vi "Continuous_Measurement_v3.vi"() -> ()   [LabVIEW 2014]
uses:
  <vilib>/Analysis/NI_AALBase.lvlib
panel:
  out "Start Timer":u32
  out "I":dbl[](array[numeric])
  out "V":dbl[](array[numeric])
  out "T":dbl[](array[numeric])
  out "File Startname":string
  in  "stop":bool
  out "I-t Graph":cluster{u32[], "I":dbl[]}(graph)
  out "V-t Graph":cluster{u32[], "V":dbl[]}(graph)
  out "V-I Graph":cluster{dbl[], dbl[]}(graph)
  in  "Meas. wait time (ms)":i32
  in  "Meas. to Avg":i32
  out "Voltage (V)":string
  in  "Current (uA)":dbl
  in  "Collect":bool
  in  "Outp. wait time (ms)":i32
  in  "2182A VISA":refnum<visa-resource-name>
  in  "Output Response":bool
  in  "Compliance (V)":dbl
  out "File Counter":i32
  out "Data Counter":i32
  in  "6221 VISA":refnum<visa-resource-name>
  in  "First Path":path
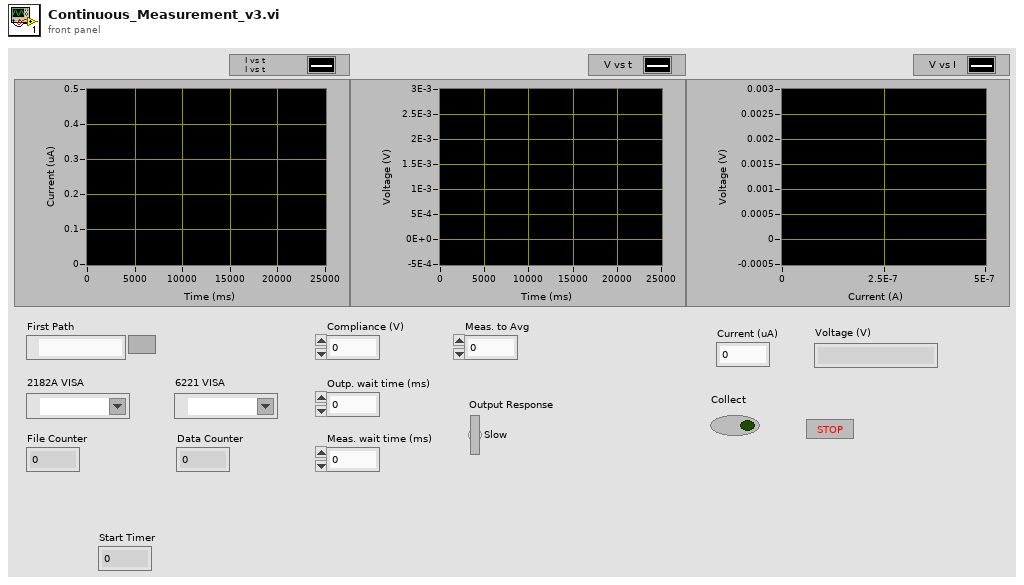
[diagram p1: front panel]
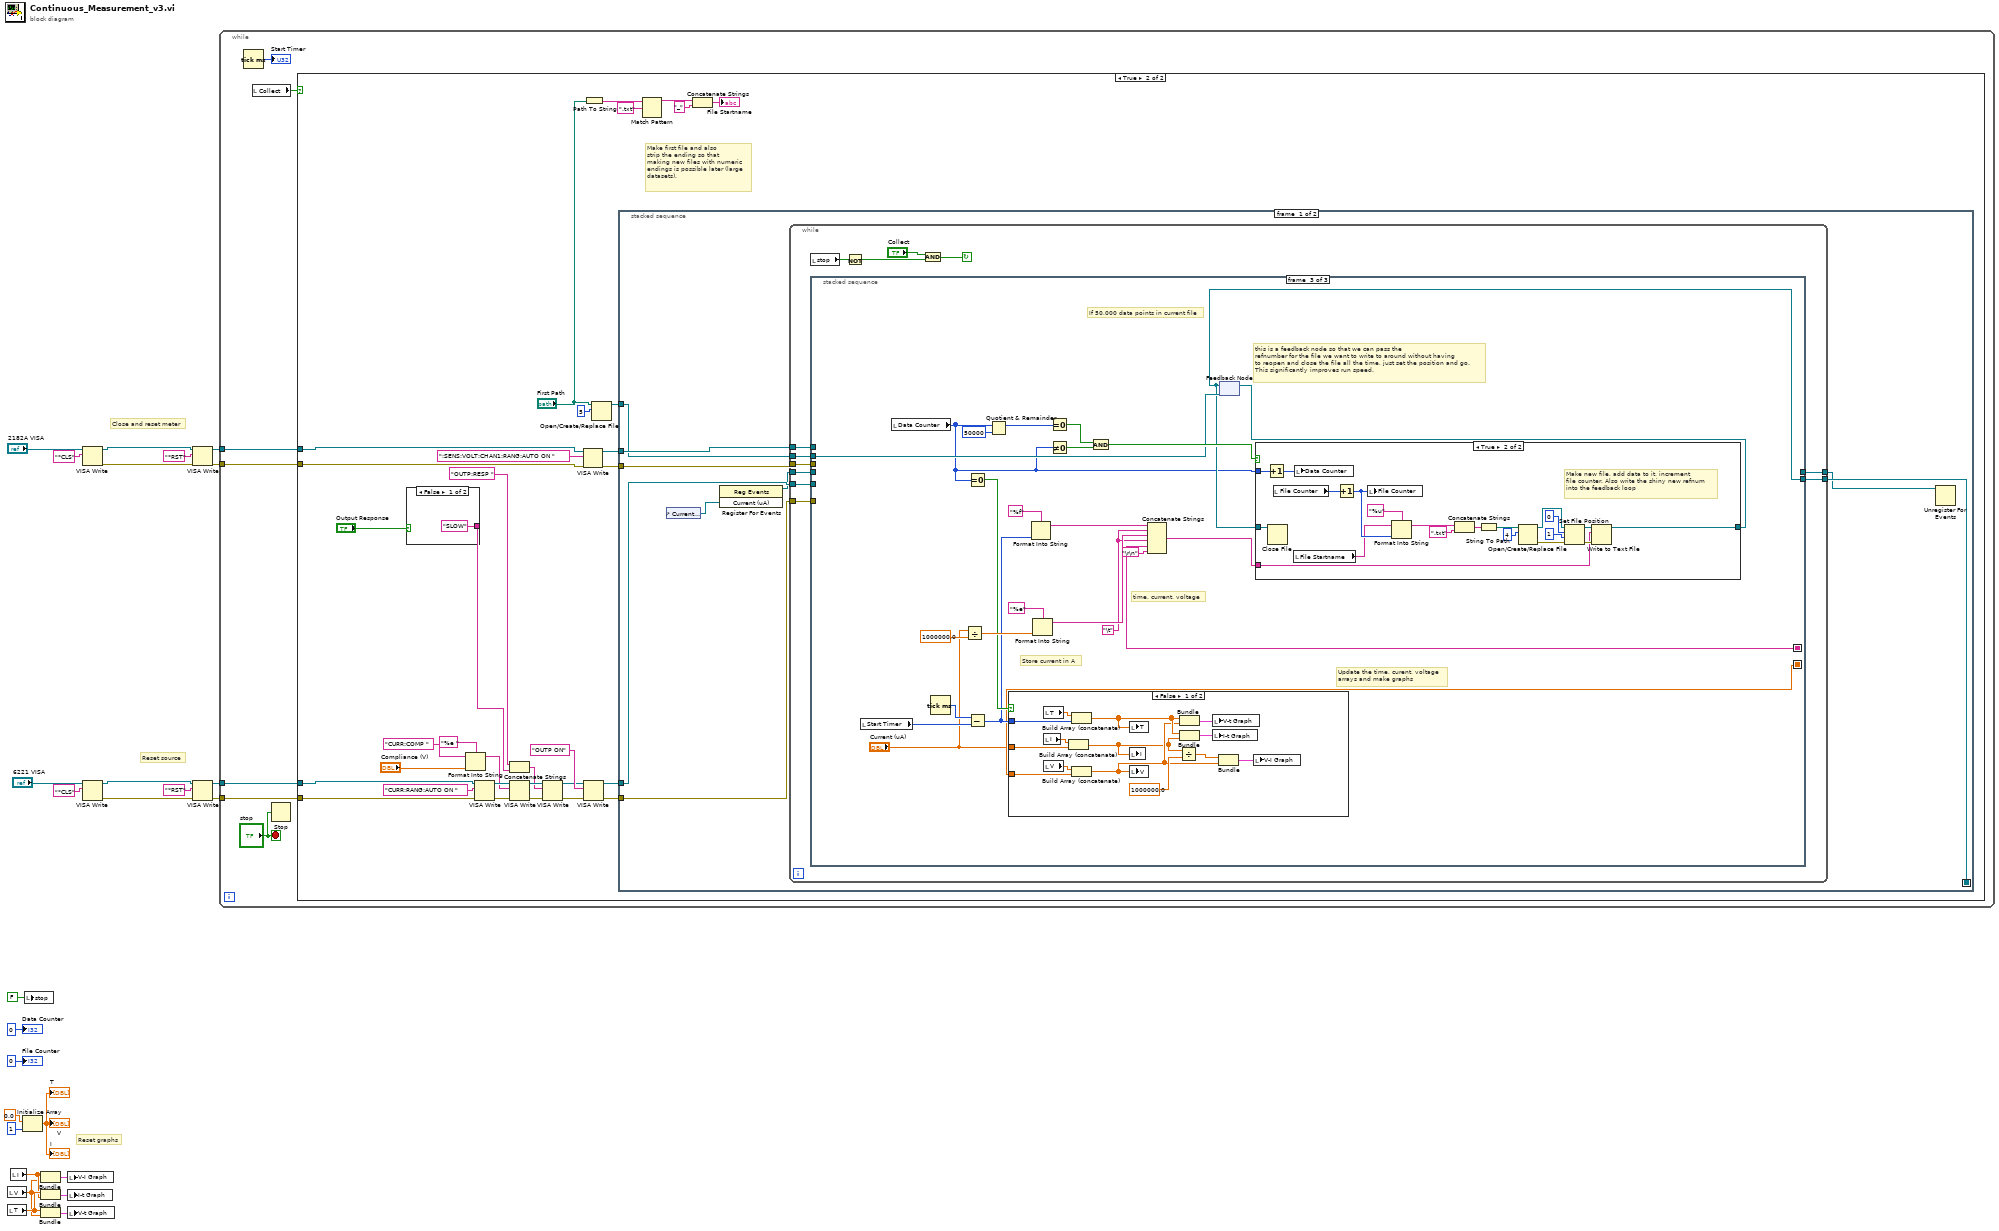
[diagram p0: block diagram]
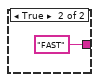
[diagram p3: hidden frame]
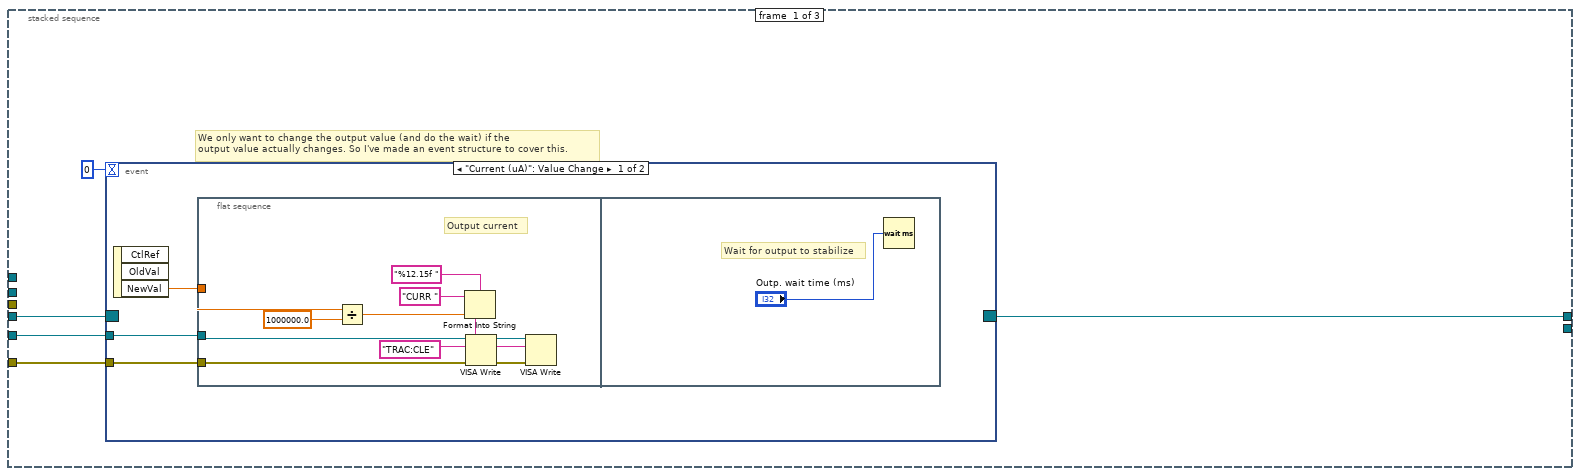
[diagram p4: hidden frame]
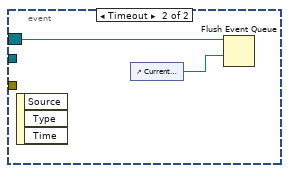
[diagram p5: hidden frame]
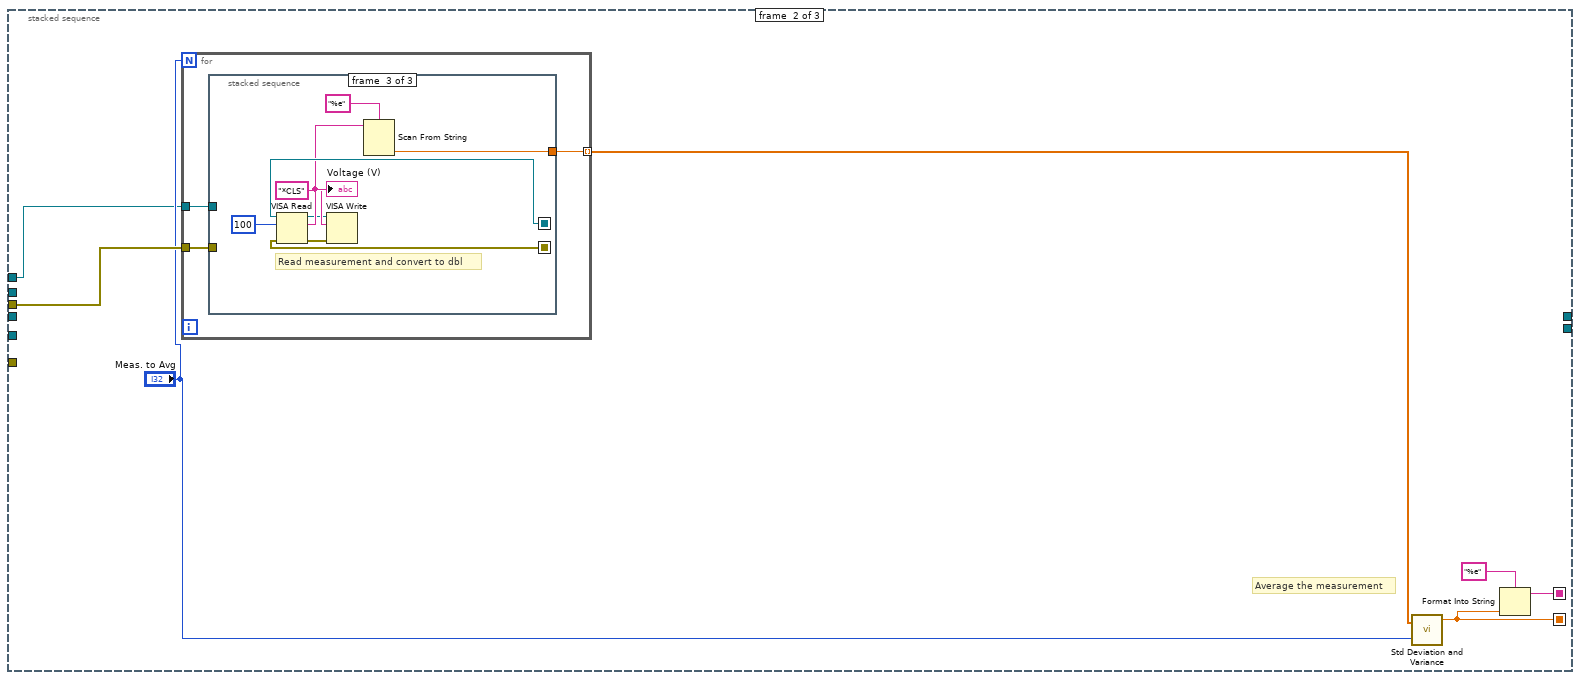
[diagram p6: hidden frame]
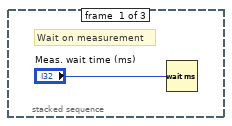
[diagram p7: hidden frame]
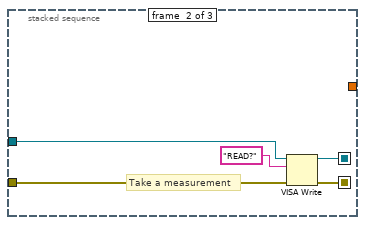
[diagram p8: hidden frame]
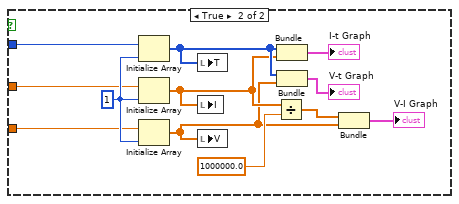
[diagram p9: hidden frame]
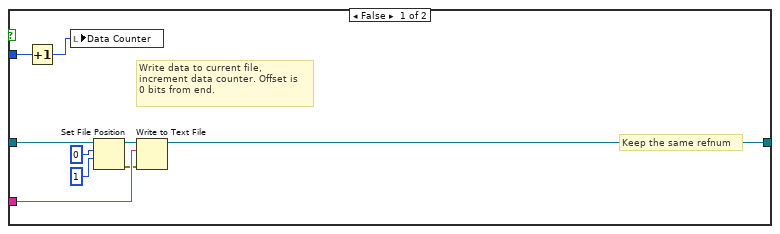
[diagram p10: hidden frame]
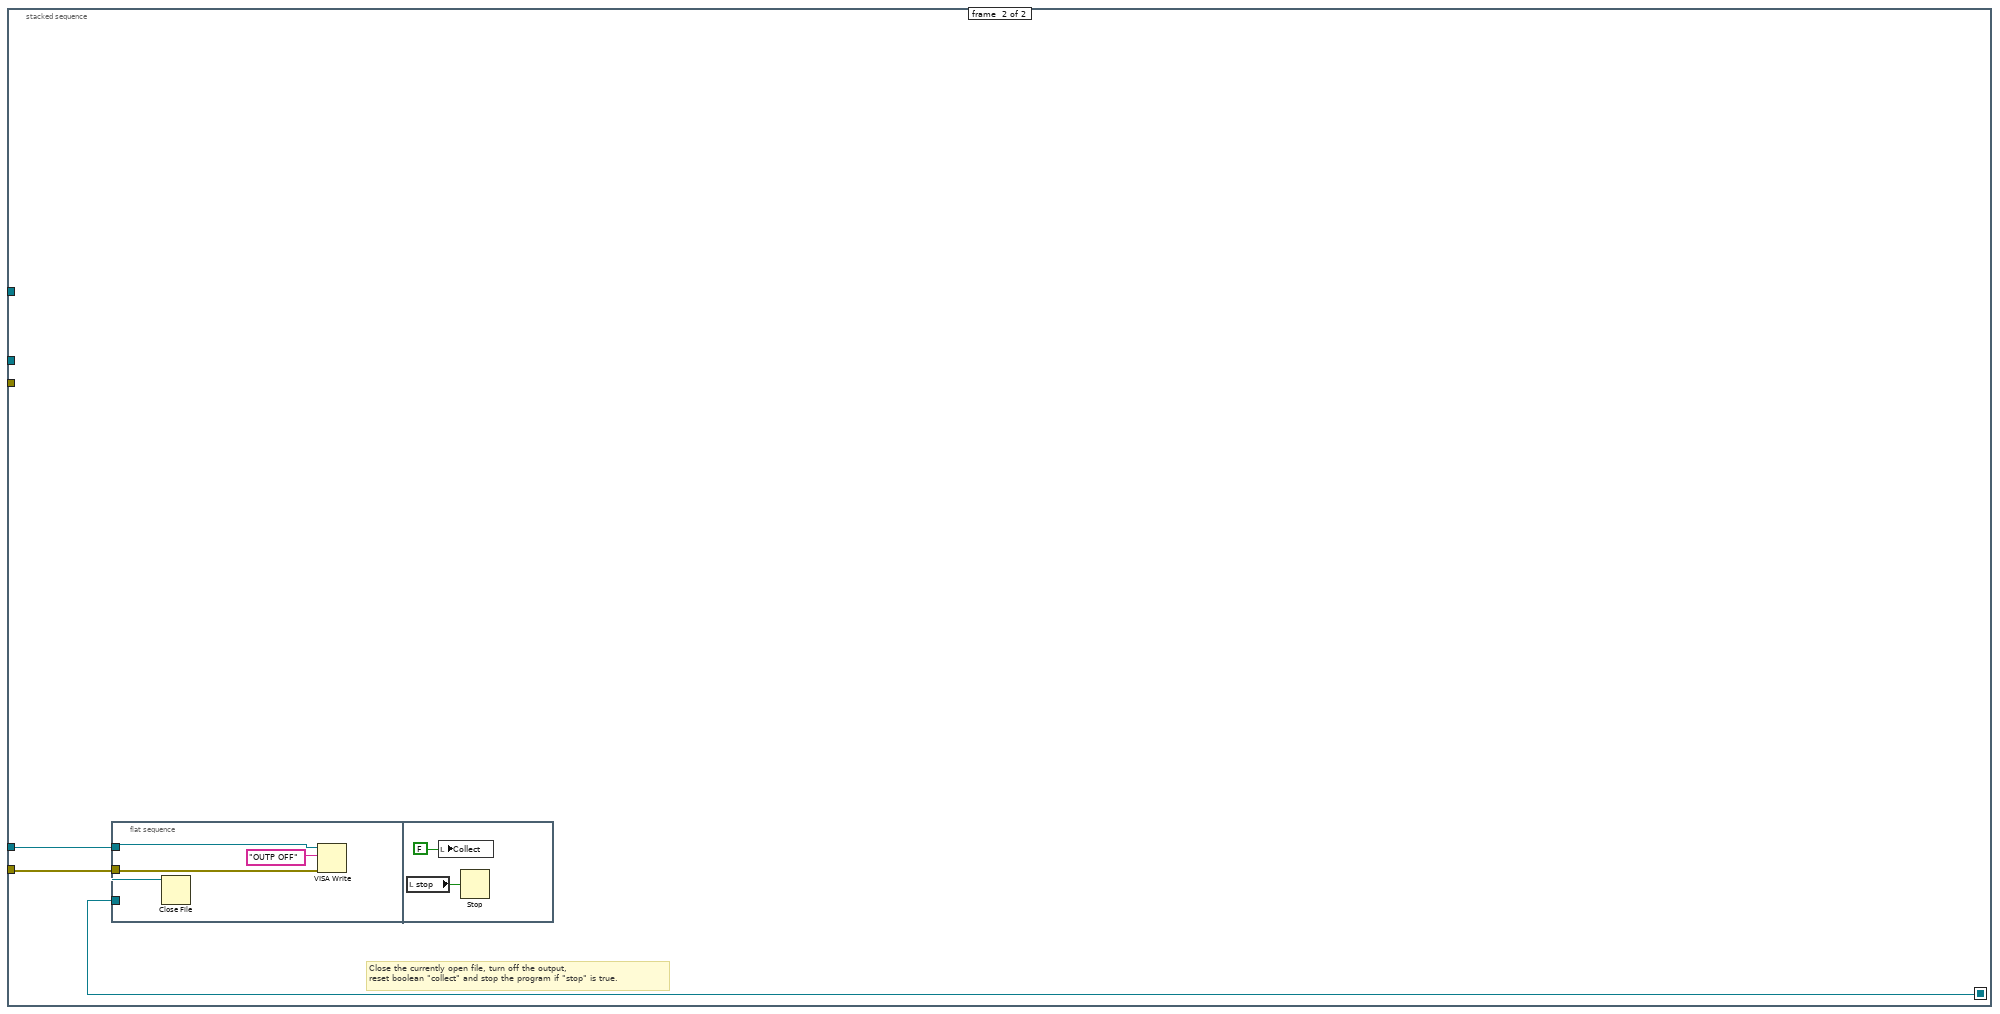
[diagram p11: hidden frame]
diagram:
  # "Reset graphs"
  # "Reset source"
  # "Close and reset meter"
  n1 = local read "V"() -> (w4:dbl[])
  n2 = local read "T"() -> (w6:dbl[])
  n3 = local read "I"() -> (w5:dbl[])
  n4 = Initialize Array(0.0, 1) -> (→"T" →"V" →"I":dbl[])
  n5 = local write "stop"(FALSE) -> ()
  n6 = Bundle("I"=w5, "V"=w4) -> (w1:cluster{"I":dbl[], "V":dbl[]})  [unwired: 1 in]
  n7 = Bundle("T"=w6, "I"=w5) -> (w3:cluster{"T":dbl[], "I":dbl[]})  [unwired: 1 in]
  n8 = Bundle("T"=w6, "V"=w4) -> (w2:cluster{"T":dbl[], "V":dbl[]})  [unwired: 1 in]
  n9 = local write "V-I Graph"(w1) -> ()
  n10 = local write "I-t Graph"(w3) -> ()
  n11 = local write "V-t Graph"(w2) -> ()
  n12 = VISA Write(VISA resource name="2182A VISA", write buffer="*CLS") -> (VISA resource name out=w18:refnum<visa-resource-name>, error out=w23:errorcluster)  [unwired: 1 in, 1 out]
  n13 = VISA Write(VISA resource name="6221 VISA", write buffer="*CLS") -> (VISA resource name out=w11:refnum<visa-resource-name>, error out=w12:errorcluster)  [unwired: 1 in, 1 out]
  n14 = VISA Write(VISA resource name=w18, write buffer="*RST", error in (no error)=w23) -> (VISA resource name out=w17:refnum<visa-resource-name>, error out=w16:errorcluster)  [unwired: 1 out]
  n15 = VISA Write(VISA resource name=w11, write buffer="*RST", error in (no error)=w12) -> (VISA resource name out=w14:refnum<visa-resource-name>, error out=w13:errorcluster)  [unwired: 1 out]
  n16 = while {
    tunnel: w17 -> [w32]
    tunnel: w16 -> [w31]
    tunnel: w14 -> [w30]
    tunnel: w13 -> [w29]
    stop <- "stop" stop-if-true
    n17 = Tick Count (ms)() -> (millisecond timer value=→"Start Timer":u32)
    n18 = local read "Collect"() -> (w33:bool)
    n19 = Stop(stop? (T)="stop") -> ()
    n20 = case shown="True" w33 {
      tunnel: w31 -> [_ w46]
      tunnel: w32 -> [_ w47]
      tunnel: w30 -> [_ w45]
      tunnel: w29 -> [_ w44]
      frame False {
      }
      frame True {
        # "Make first file and also\nstrip the ending so that\nmaking new files with numeric\nendings is possible later (large\ndatasets)."
        n21 = case shown="False" "Output Response" {
          tunnel: ["SLOW" "FAST"] -> w57
          frame False {
          }
          frame True {
          }
        }
        n22 = Format Into String(format string="%e ", initial string="CURR:COMP ", "Compliance (V)") -> (resulting string=w55:string)  [unwired: 1 in, 1 out]
        n23 = VISA Write(VISA resource name=w45, write buffer="CURR:RANG:AUTO ON ", error in (no error)=w44) -> (VISA resource name out=w60:refnum<visa-resource-name>, error out=w61:errorcluster)  [unwired: 1 out]
        n24 = Concatenate Strings("OUTP:RESP ", w57) -> (w59:string)
        n25 = VISA Write(VISA resource name=w60, write buffer=w55, error in (no error)=w61) -> (VISA resource name out=w63:refnum<visa-resource-name>, error out=w62:errorcluster)  [unwired: 1 out]
        n26 = VISA Write(VISA resource name=w63, write buffer=w59, error in (no error)=w62) -> (VISA resource name out=w51:refnum<visa-resource-name>, error out=w50:errorcluster)  [unwired: 1 out]
        n27 = VISA Write(VISA resource name=w47, write buffer=":SENS:VOLT:CHAN1:RANG:AUTO ON ", error in (no error)=w46) -> (VISA resource name out=w49:refnum<visa-resource-name>, error out=w48:errorcluster)  [unwired: 1 out]
        n28 = VISA Write(VISA resource name=w51, write buffer="OUTP ON", error in (no error)=w50) -> (VISA resource name out=w65:refnum<visa-resource-name>, error out=w64:errorcluster)  [unwired: 1 out]
        n29 = Path To String(path="First Path") -> (string=w42:string)
        n30 = Open/Create/Replace File(file path (use dialog)="First Path", operation (0:open)=5) -> (refnum out=w37:refnum<file>)  [unwired: 4 in, 2 out]
        n31 = stacked-sequence {
          seq-local: [w72 _] -> [_ w217]
          tunnel: w64 -> [w77 w218]
          tunnel: w48 -> [w76 _]
          tunnel: w65 -> [w75 w219]
          tunnel: w49 -> [w74 _]
          tunnel: w37 -> [w73 _]
          frame #0 {
            n32 = control-ref of="Current (uA)"() -> (w71:refnum<vi>)
            n33 = register-events(w71) -> (reference out=w70:refnum<event-registration>)  [unwired: 2 in, 1 out]
            n34 = while {
              tunnel: w77 -> [w89]
              tunnel: w76 -> [w79]
              tunnel: w75 -> [w85]
              tunnel: w74 -> [w78]
              tunnel: w73 -> [w83]
              tunnel: [w82] -> w72
              tunnel: w70 -> [w81]
              tunnel: [w80] -> w69
              stop <- w86 continue-if-true
              n35 = local read "stop"() -> (w84:bool)
              n36 = stacked-sequence {
                seq-local: [_ w114 _] -> [_ _ w149]
                seq-local: [_ w112 _] -> [_ _ w140]
                tunnel: w89 -> [w93 _ _]
                tunnel: w79 -> [_ w118 _]
                tunnel: w85 -> [w94 _ _]
                tunnel: w78 -> [_ w113 _]
                tunnel: w83 -> [_ _ w145]
                tunnel: [_ _ w143] -> w82
                tunnel: w81 -> [w92 _ _]
                tunnel: [w91 _ _] -> w80
                frame #0 {
                  # "We only want to change the output value (and do the wait) if the\noutput value actually changes. So I've made an event structure to cover this."
                  n37 = event shown="[0] \"Current (uA)\": Value Change" {
                    selector: w92 -> [_ w111]
                    dyn-events: [_ _] -> w91
                    timeout: 0 -> [_ _]
                    tunnel: w94 -> [w96 _]
                    tunnel: w93 -> [w95 _]
                    event "Current (uA)": Value Change {
                      n38 = event-data() -> ("NewVal"=w97:dbl)  [unwired: 1 in, 2 out]
                      n39 = flat-sequence {
                        tunnel: w97 -> [w100]
                        tunnel: w96 -> [w99]
                        tunnel: w95 -> [w98]
                        frame #0 {
                          # "Output current"
                          n40 = Divide(x=w100, y=1000000.0) -> (x/y=w103:dbl)
                          n41 = Format Into String(format string="%12.15f ", initial string="CURR ", w103) -> (resulting string=w105:string)  [unwired: 1 in, 1 out]
                          n42 = VISA Write(VISA resource name=w99, write buffer="TRAC:CLE", error in (no error)=w98) -> (VISA resource name out=w102:refnum<visa-resource-name>, error out=w107:errorcluster)  [unwired: 1 out]
                          n43 = VISA Write(VISA resource name=w102, write buffer=w105, error in (no error)=w107) -> ()  [unwired: 3 out]
                        }
                        frame #1 {
                          # "Wait for output to stabilize"
                          n44 = Wait (ms)(milliseconds to wait="Outp. wait time (ms)") -> ()  [unwired: 1 out]
                        }
                      }
                    }
                    event Timeout {
                      n45 = event-data() -> ()  [unwired: 1 in, 3 out]
                      n46 = control-ref of="Current (uA)"() -> (w110:refnum<vi>)
                      n47 = Flush Event Queue(0:w111, 2:w110) -> ()  [unwired: 4 in, 3 out]
                    }
                  }
                }
                frame #1 {
                  # "Average the measurement"
                  n48 = for {
                    N: "Meas. to Avg" -> [_]
                    tunnel: w118 -> [w121]
                    tunnel: [w120] -> w117 mode=indexing
                    tunnel: w113 -> [w119]
                    n49 = stacked-sequence {
                      seq-local: [_ w125 _] -> [_ _ w135]
                      seq-local: [_ w123 _] -> [_ _ w132]
                      tunnel: w121 -> [_ w126 _]
                      tunnel: [_ _ w133] -> w120
                      tunnel: w119 -> [_ w124 _]
                      frame #0 {
                        # "Wait on measurement"
                        n50 = Wait (ms)(milliseconds to wait="Meas. wait time (ms)") -> ()  [unwired: 1 out]
                      }
                      frame #1 {
                        # "Take a measurement"
                        n51 = VISA Write(VISA resource name=w124, write buffer="READ?", error in (no error)=w126) -> (VISA resource name out=w123:refnum<visa-resource-name>, error out=w125:errorcluster)  [unwired: 1 out]
                      }
                      frame #2 {
                        # "Read measurement and convert to dbl"
                        n52 = VISA Read(VISA resource name=w132, byte count=100, error in (no error)=w135) -> (VISA resource name out=w129:refnum<visa-resource-name>, read buffer=w131:string, error out=w128:errorcluster)  [unwired: 1 out]
                        "Voltage (V)" <- w131
                        n53 = VISA Write(VISA resource name=w129, write buffer="*CLS", error in (no error)=w128) -> ()  [unwired: 3 out]
                        n54 = Scan From String(format string="%e", input string=w131) -> (output 1=w133:dbl)  [unwired: 3 in, 3 out]
                      }
                    }
                  }
                  n55 = call <vilib>:"Std Deviation and Variance.vi"("X"=w117, "Weighting (Sample)"="Meas. to Avg") -> ("mean"=w112:dbl)  [unwired: 2 out]
                  n56 = Format Into String(format string="%e", w112) -> (resulting string=w114:string)  [unwired: 2 in, 1 out]
                }
                frame #2 {
                  w156 = "\t"
                  # "Store current in A"
                  # "Update the time, curent, voltage\narrays and make graphs"
                  # "this is a feedback node so that we can pass the\nrefnumber for the file we want to write to around without having\nto reopen and close the file all the time, just set the position and go. \nThis significantly improves run speed."
                  # "time, current, voltage"
                  # "If 50,000 data points in current file"
                  n57 = local read "Start Timer"() -> (w139:u32)
                  n58 = local read "Data Counter"() -> (w138:i32)
                  n59 = Tick Count (ms)() -> (millisecond timer value=w161:u32)
                  n60 = Divide(x="Current (uA)", y=1000000.0) -> (x/y=w148:dbl)
                  n61 = Equal To 0?(x=w138) -> (x = 0?=w142:bool)
                  n62 = Subtract(x=w161, y=w139) -> (x-y=w141:u32)
                  n63 = Quotient & Remainder(x=w138, y=50000) -> (x-y*floor(x/y)=w146:i32)  [unwired: 1 out]
                  n64 = case shown="False" w142 {
                    tunnel: w141 -> [w174 w181]
                    tunnel: w140 -> [w170 w179]
                    tunnel: "Current (uA)" -> [w171 w180]
                    frame False {
                      n65 = local read "T"() -> (w175:dbl[])
                      n66 = local read "I"() -> (w173:dbl[])
                      n67 = local read "V"() -> (w172:dbl[])
                      n68 = Build Array (concatenate)(w173, w171) -> (w162:dbl[])
                      n69 = Build Array (concatenate)(w175, w174) -> (w164:dbl[])
                      n70 = Build Array (concatenate)(w172, w170) -> (w163:dbl[])
                      n71 = local write "T"(w164) -> ()
                      n72 = local write "I"(w162) -> ()
                      n73 = local write "V"(w163) -> ()
                      n74 = Divide(x=w162, y=1000000.0) -> (x/y=w166:dbl[])
                      n75 = Bundle(w164, w163) -> (w168:cluster{dbl[], dbl[]})  [unwired: 1 in]
                      n76 = Bundle(w164, w162) -> (w167:cluster{dbl[], dbl[]})  [unwired: 1 in]
                      n77 = local write "V-t Graph"(w168) -> ()
                      n78 = local write "I-t Graph"(w167) -> ()
                      n79 = Bundle(w166, w163) -> (w169:cluster{dbl[], dbl[]})  [unwired: 1 in]
                      n80 = local write "V-I Graph"(w169) -> ()
                    }
                    frame True {
                      w182 = 1
                      n81 = Initialize Array(w181, w182) -> (w178:u32[])
                      n82 = Initialize Array(w180, w182) -> (w177:dbl[])
                      n83 = Initialize Array(w179, w182) -> (w176:dbl[])
                      n84 = local write "T"(w178) -> ()
                      n85 = local write "I"(w177) -> ()
                      n86 = local write "V"(w176) -> ()
                      n87 = Divide(x=w177, y=1000000.0) -> (x/y=w186:dbl[])
                      n88 = Bundle(w178, w177) -> (→"I-t Graph":cluster{u32[], dbl[]})  [unwired: 1 in]
                      n89 = Bundle(w178, w176) -> (→"V-t Graph":cluster{u32[], dbl[]})  [unwired: 1 in]
                      n90 = Bundle(w186, w176) -> (→"V-I Graph":cluster{dbl[], dbl[]})  [unwired: 1 in]
                    }
                  }
                  n91 = Format Into String(format string="%f", w141) -> (resulting string=w159:string)  [unwired: 2 in, 1 out]
                  n92 = Format Into String(format string="%e", w148) -> (resulting string=w157:string)  [unwired: 2 in, 1 out]
                  n93 = Equal To 0?(x=w146) -> (x = 0?=w153:bool)
                  n94 = Not Equal To 0?(x=w138) -> (x != 0?=w152:bool)
                  n95 = And(x=w153, y=w152) -> (x .and. y?=w151:bool)
                  n96 = Concatenate Strings(w159, w156, w157, w156, w149, "\r\n") -> (w150:string)
                  n97 = feedback #1(w145) -> (w143:refnum<file>)
                  n98 = case shown="True" w151 {
                    tunnel: w150 -> [w193 w206]
                    tunnel: [w191 w205] -> w144
                    tunnel: w143 -> [w190 w216]
                    tunnel: w138 -> [w188 w198]
                    frame False {
                      # "Keep the same refnum"
                      # "Write data to current file,\nincrement data counter. Offset is\n0 bits from end."
                      n99 = Increment(x=w188) -> (x+1=w189:i32)
                      n100 = local write "Data Counter"(w189) -> ()
                      n101 = Set File Position(offset (in bytes) (0)=0, refnum=w190, from (0:start)=1) -> (refnum out=w194:refnum<file>, error out=w192:errorcluster)  [unwired: 1 in]
                      n102 = Write to Text File(file (use dialog)=w194, text=w193, error in=w192) -> (refnum out=w191:refnum<file>)  [unwired: 1 in, 2 out]
                    }
                    frame True {
                      # "Make new file, add data to it, increment\nfile counter. Also write the shiny new refnum\ninto the feedback loop"
                      n103 = Increment(x=w198) -> (x+1=w199:i32)
                      n104 = Close File(refnum=w216) -> ()  [unwired: 1 in, 2 out]
                      n105 = local read "File Counter"() -> (w204:i32)
                      n106 = local read "File Startname"() -> (w197:string)
                      n107 = local write "Data Counter"(w199) -> ()
                      n108 = Increment(x=w204) -> (x+1=w200:i32)
                      n109 = local write "File Counter"(w200) -> ()
                      n110 = Format Into String(format string="%u", initial string=w197, w200) -> (resulting string=w215:string)  [unwired: 1 in, 1 out]
                      n111 = Concatenate Strings(w215, ".txt") -> (w211:string)
                      n112 = String To Path(string=w211) -> (path=w213:path)
                      n113 = Open/Create/Replace File(file path (use dialog)=w213, operation (0:open)=u16 4) -> (refnum out=w203:refnum<file>, error out=w202:errorcluster)  [unwired: 4 in, 1 out]
                      n114 = Set File Position(offset (in bytes) (0)=i64 0, refnum=w203, from (0:start)=u16 1, error in=w202) -> (refnum out=w209:refnum<file>, error out=w210:errorcluster)
                      n115 = Write to Text File(file (use dialog)=w209, text=w206, error in=w210) -> (refnum out=w205:refnum<file>)  [unwired: 1 in, 2 out]
                    }
                  }
                  n116 = feedback-in #1(w144) -> ()
                }
              }
              n117 = Not(x=w84) -> (.not. x?=w87:bool)
              n118 = And(x="Collect", y=w87) -> (x .and. y?=w86:bool)
            }
            n119 = Unregister For Events(event registration refnum=w69) -> ()  [unwired: 1 in, 1 out]
          }
          frame #1 {
            # "Close the currently open file, turn off the output,\nreset boolean \"collect\" and stop the program if \"stop\" is true."
            n120 = flat-sequence {
              tunnel: w219 -> [w222]
              tunnel: w218 -> [w221]
              tunnel: w217 -> [w220]
              frame #0 {
                n121 = Close File(refnum=w220) -> ()  [unwired: 1 in, 2 out]
                n122 = VISA Write(VISA resource name=w222, write buffer="OUTP OFF", error in (no error)=w221) -> ()  [unwired: 3 out]
              }
              frame #1 {
                n123 = local read "stop"() -> (w225:bool)
                n124 = local write "Collect"(FALSE) -> ()
                n125 = Stop(stop? (T)=w225) -> ()
              }
            }
          }
        }
        n126 = Match Pattern(string=w42, regular expression=".txt") -> (before substring=w36:string)  [unwired: 1 in, 3 out]
        n127 = Concatenate Strings(w36, "_") -> (→"File Startname":string)
      }
    }
  }
  "Data Counter" <- 0
  "File Counter" <- 0
